vi "Load Targets from Disc.vi"(8 "error in (no error)":errorcluster, 9 "Unhandled Path":path, 10 "External Path":path, 11 "Internal Path":path) -> (0 "error out":errorcluster, 1 "Unhandled Dependencies":string[](array[string]), 2 "External Target Map":map{string, string}(c390), 3 "Internal Target Map":map{string, string}(c390))   [LabVIEW 2019, in "Project.Dependencies Finder.lvlib" / "Dependency Source.lvclass"]
doc: "Load dependency source data from disc for the given paths."
uses:
  Dependency Source.lvclass
  <vilib>/Utility/file.llb/Read Delimited Spreadsheet (string).vi
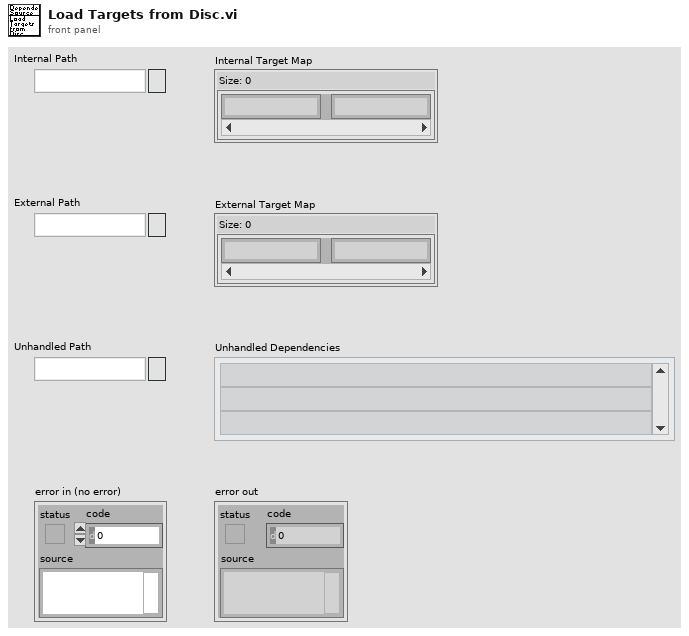
[diagram p1: front panel]
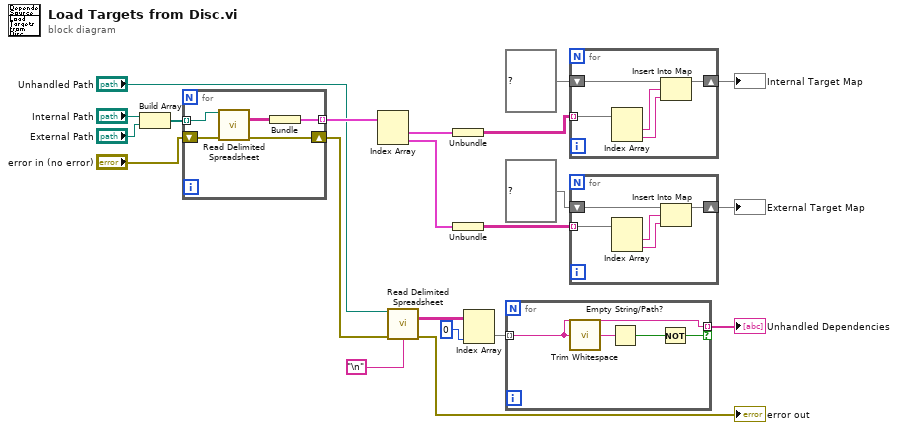
[diagram p0: block diagram]
diagram:
  n1 = Build Array("Internal Path", "External Path") -> (w19:path[])
  n2 = for {
    tunnel: w19 -> [w26] mode=indexing
    shift-right: [w24] -> w2
    shift-left: "error in (no error)" -> [w25]
    tunnel: [w22] -> w17 mode=indexing
    n3 = call-poly <vilib>:"Read Delimited Spreadsheet.vi"("file path (dialog if empty)"=w26, "error in (no error)"=w25) -> ("all rows"=w23:string[][], "error out"=w24:errorcluster)  [unwired: 8 in, 4 out]
    n4 = Bundle("all rows"=w23) -> (w22:cluster{"all rows":string[][]})  [unwired: 1 in]
  }
  n5 = Index Array(array=w17) -> (element #1=w16:cluster{"all rows":string[][]}, element #2=w15:cluster{"all rows":string[][]})  [unwired: 2 in]
  n6 = call-poly <vilib>:"Read Delimited Spreadsheet.vi"("file path (dialog if empty)"="Unhandled Path", "error in (no error)"=w2, "delimiter (\\t)"="\n") -> ("all rows"=w4:string[][], "error out"=→"error out":errorcluster)  [unwired: 7 in, 4 out]
  n7 = Unbundle(w16) -> ("all rows"=w14:string[][])
  n8 = Unbundle(w15) -> ("all rows"=w9:string[][])
  n9 = Index Array(array=w4, index (col)=0 ("disabled index (col)")) -> (element=w7:string[])  [unwired: 1 in]
  n10 = for {
    tunnel: w7 -> [w28] mode=indexing
    tunnel: [w28] -> w6 mode=indexing if=w27
    n11 = call <vilib>:"Trim Whitespace.vi"("string"=w28) -> ("trimmed string"=w30:string)  [unwired: 1 in]
    n12 = Empty String/Path?(string/path=w30) -> (empty?=w29:bool)
    n13 = Not(x=w29) -> (.not. x?=w27:bool)
  }
  "Unhandled Dependencies" <- w6
  n14 = for {
    shift-right: [w33] -> w12
    shift-left: map{string, string} {} ("Internal Target Map") -> [w34]
    tunnel: w14 -> [w35] mode=indexing
    n15 = Index Array(array=w35) -> (element #1=w32:string, element #2=w31:string)  [unwired: 2 in]
    n16 = Insert Into Map(map in=w34, key=w32, value=w31) -> (map out=w33:map{string, string})  [unwired: 2 out]
  }
  "Internal Target Map" <- w12
  n17 = for {
    shift-right: [w38] -> w10
    shift-left: map{string, string} {} ("External Target Map") -> [w39]
    tunnel: w9 -> [w40] mode=indexing
    n18 = Index Array(array=w40) -> (element #1=w37:string, element #2=w36:string)  [unwired: 2 in]
    n19 = Insert Into Map(map in=w39, key=w37, value=w36) -> (map out=w38:map{string, string})  [unwired: 2 out]
  }
  "External Target Map" <- w10
